vi "Obtain Broadcast Events.vi"(8 "error in":errorcluster, 10 "Create New? (F)":bool) -> (0 "error out":errorcluster, 2 "RT Acquisition Engine Broadcast Events":T1)   [LabVIEW 2021, in "RT Acquisition Engine.lvlib"]
doc: "This VI Obtains/Creates the Broadcast events that will be used for other modules to register to receive messages from the module that owns this VI.\n\n<b>NOTE</b>: The contents of this VI are automatically generated and modified by the <b>Tools > DQMH Consortium > DQMH</b> utilities. Consider using those utilities instead of making your own modifications to this VI.\n_____\nBased on DQMH Project Template 7.0.1.1316."
uses:
  RT Acquisition Engine.lvlib
  Broadcast Events--cluster.ctl
  Did Init Argument--cluster.ctl
  Status Updated Argument--cluster.ctl
  Error Reported Argument--cluster.ctl
  Stop Argument--cluster.ctl
  Get Module Execution Status Argument--cluster.ctl
  RT Connection Status Argument--cluster.ctl
  Hardware Info (Reply Payload)--cluster.ctl
  DO Data's Argument--cluster.ctl
  Host-Control's/DIO Data's from RT.ctl
  AI-Info Argument--cluster.ctl
  Host-Control's/AI-Data from RT.ctl
  Logging Completed Argument--cluster.ctl
panel:
  # "NOTE: The contents of this VI are automatically generated and modified by the Tools > DQMH Consortium > DQMH utilities. Consider using those utilities instead of making your own modifications to this VI."
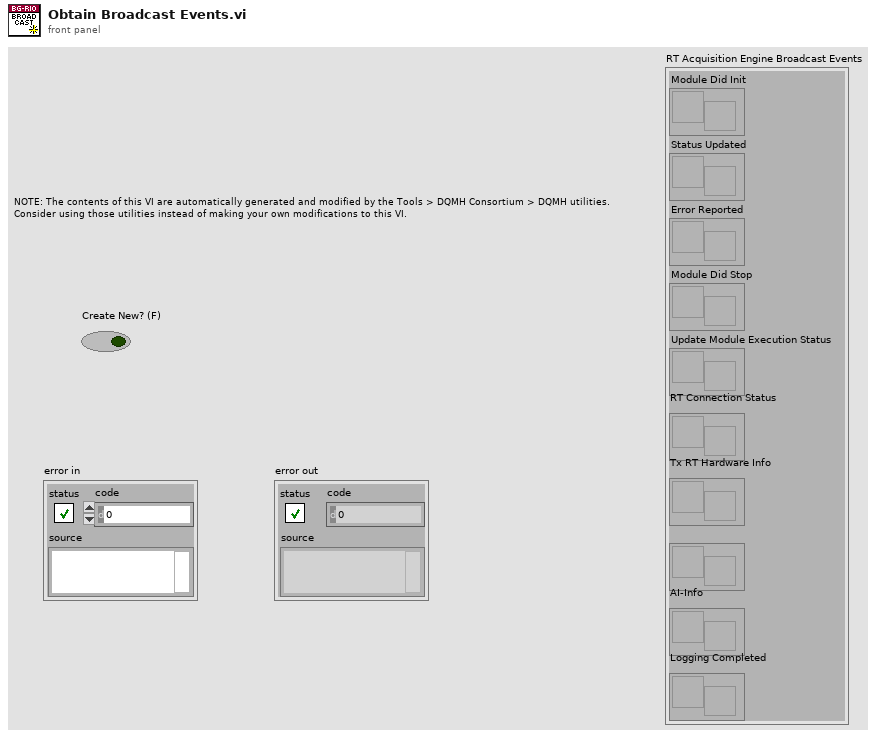
[diagram p1: front panel]
types:
  T1 = typedef "RT Acquisition Engine.lvlib/Broadcast Events--cluster.ctl" = cluster{"Module Did Init":refnum<user-event>, "Status Updated":refnum<user-event>, "Error Reported":refnum<user-event>, "Module Did Stop":refnum<user-event>, "Update Module Execution Status":refnum<user-event>, "RT Connection Status":refnum<user-event>, "Tx RT Hardware Info":refnum<user-event>, "DO Data's":refnum<user-event>, "AI-Info":refnum<user-event>, "Logging Completed":refnum<user-event>}
  T2 = typedef "RT Acquisition Engine.lvlib/Logging Completed Argument--cluster.ctl" = cluster{"Module ID":i32, "Logging Completed?":bool}
  T3 = typedef "RT Acquisition Engine.lvlib/AI-Info Argument--cluster.ctl" = cluster{"Module ID":i32, "AI-Info":T4}
  T4 = typedef "AI-Data from RT.ctl" = cluster{"Channel Name's":string[], "Channel Data's":dbl[], "Date & Time":string}
  T5 = typedef "RT Acquisition Engine.lvlib/DO Data's Argument--cluster.ctl" = cluster{"Module ID":i32, "DO Data's":T6}
  T6 = typedef "DIO Data's from RT.ctl" = cluster{"Channels":string[], "Data":bool[], "Time":string}
  T7 = typedef "RT Acquisition Engine.lvlib/Hardware Info (Reply Payload)--cluster.ctl" = cluster{"Module ID":i32, "Hardware Information":variant, "error":errorcluster}
  T8 = typedef "RT Acquisition Engine.lvlib/RT Connection Status Argument--cluster.ctl" = cluster{"Module ID":i32, "RT Connection Status?":bool}
  T9 = typedef "RT Acquisition Engine.lvlib/Get Module Execution Status Argument--cluster.ctl" = cluster{"Module ID":i32, "Running?":bool}
  T10 = typedef "RT Acquisition Engine.lvlib/Stop Argument--cluster.ctl" = cluster{"Module ID":i32, "Origin":string, "Exit via Stop Module Req?":bool, "Wait for Module to stop?":bool}
  T11 = typedef "RT Acquisition Engine.lvlib/Error Reported Argument--cluster.ctl" = cluster{"Error":errorcluster, "Additional Information":string, "Module ID":i32, "Module Name":string}
  T12 = typedef "RT Acquisition Engine.lvlib/Status Updated Argument--cluster.ctl" = cluster{"Status":string, "Module ID":i32}
  T13 = typedef "RT Acquisition Engine.lvlib/Did Init Argument--cluster.ctl" = cluster{"Init?":bool, "Info":string, "Module ID":i32}
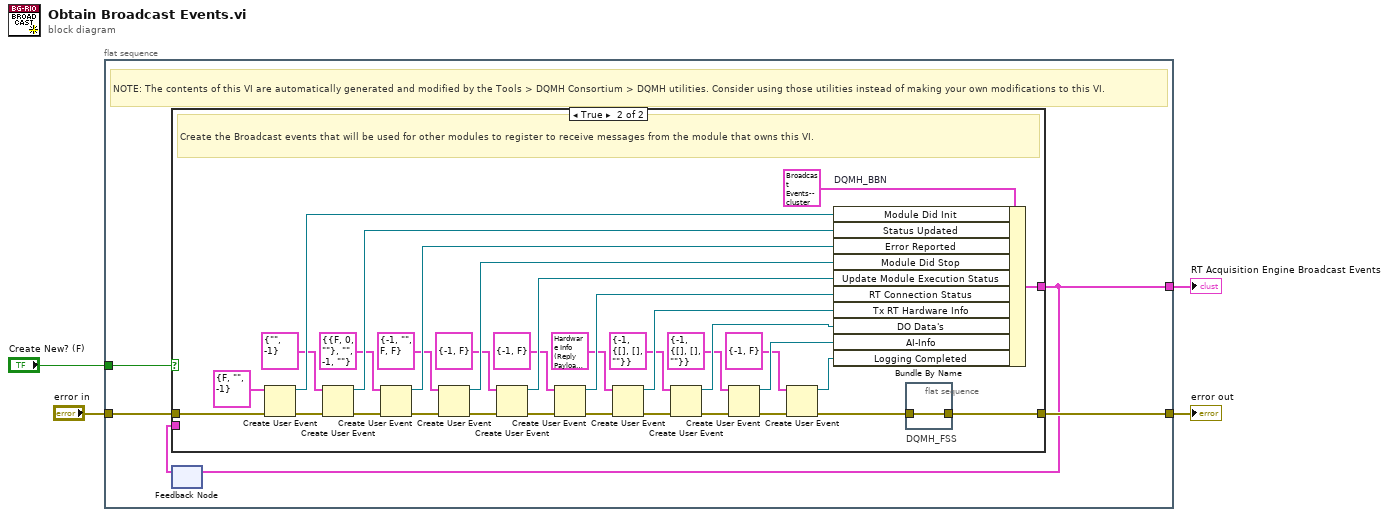
[diagram p0: block diagram]
diagram:
  n1 = flat-sequence {
    tunnel: [w9] -> w4
    tunnel: "error in" -> [w8]
    tunnel: [w6] -> w2
    tunnel: "Create New? (F)" -> [w5]
    frame #0 {
      # "NOTE: The contents of this VI are automatically generated and modified by the Tools > DQMH Consortium > DQMH utilities. Consider using those utilities instead of making your own modifications to this VI."
      n2 = feedback #1() -> (w7:T1)  [unwired: 1 in]
      n3 = case shown="True" w5 {
        tunnel: [w10 w30] -> w9
        tunnel: w8 -> [w10 w45]
        tunnel: [w11 w42] -> w6
        tunnel: w7 -> [w11 _]
        frame False {
          # "Obtain the Broadcast events that were created in a previous call to this VI."
        }
        frame True {
          # "Create the Broadcast events that will be used for other modules to register to receive messages from the module that owns this VI."
          n4 = Create User Event(user event datatype=T13 {"Init?"=FALSE, "Info"="", "Module ID"=-1} ("Did Init Argument"), error in=w45) -> (user event=w43:refnum<user-event>, error out=w40:errorcluster)
          n5 = Create User Event(user event datatype=T12 {"Status"="", "Module ID"=-1} ("Status Updated Argument"), error in=w40) -> (user event=w37:refnum<user-event>, error out=w39:errorcluster)
          n6 = Create User Event(user event datatype=T11 {"Error"={"status"=FALSE, "code"=0, "source"=""}, "Additional Information"="", "Module ID"=-1, "Module Name"=""} ("Error Reported Argument"), error in=w39) -> (user event=w34:refnum<user-event>, error out=w36:errorcluster)
          n7 = Create User Event(user event datatype=T10 {"Module ID"=-1, "Origin"="", "Exit via Stop Module Req?"=FALSE, "Wait for Module to stop?"=FALSE} ("Stop Argument"), error in=w36) -> (user event=w32:refnum<user-event>, error out=w31:errorcluster)
          n8 = Create User Event(user event datatype=T9 {"Module ID"=-1, "Running?"=FALSE} ("Get Module Execution Status Argument"), error in=w31) -> (user event=w28:refnum<user-event>, error out=w29:errorcluster)
          n9 = Create User Event(user event datatype=T8 {"Module ID"=-1, "RT Connection Status?"=FALSE} ("RT Connection Status Argument"), error in=w29) -> (user event=w25:refnum<user-event>, error out=w26:errorcluster)
          n10 = Create User Event(user event datatype=T7 {"Module ID"=-1, "Hardware Information"=variant(cluster{"Serial Hardware Info JSON Format":cluster{"Command":string, "SubCmd":string, "Channel":string[]}, "Hardware Info JSON Format":cluster{"Command":string, "SubCmd":string, "Input":string[], "Output":string[]}, "Hardware Info JSON Format":cluster{"Command":string, "SubCmd":string, "Input":string[], "Output":string[]}, "Ethernet IP Address JSON Format":cluster{"Command":string, "SubCmd":string, "IP":string[]}} {"Serial Hardware Info JSON Format"={"Command"="", "SubCmd"="", "Channel"=[]}, "Hardware Info JSON Format"={"Command"="", "SubCmd"="", "Input"=[], "Output"=[]}, "Hardware Info JSON Format"={"Command"="", "SubCmd"="", "Input"=[], "Output"=[]}, "Ethernet IP Address JSON Format"={"Command"="", "SubCmd"="", "IP"=[]}}), "error"={"status"=FALSE, "code"=0, "source"=""}} ("Hardware Info (Reply Payload)"), error in=w26) -> (user event=w22:refnum<user-event>, error out=w23:errorcluster)
          n11 = Create User Event(user event datatype=T5 {"Module ID"=-1, "DO Data's"={"Channels"=[], "Data"=[], "Time"=""}} ("DO Data's Argument"), error in=w23) -> (user event=w19:refnum<user-event>, error out=w20:errorcluster)
          n12 = Create User Event(user event datatype=T3 {"Module ID"=-1, "AI-Info"={"Channel Name's"=[], "Channel Data's"=[], "Date & Time"=""}} ("AI-Info Argument"), error in=w20) -> (user event=w16:refnum<user-event>, error out=w17:errorcluster)
          n13 = Create User Event(user event datatype=T2 {"Module ID"=-1, "Logging Completed?"=FALSE} ("Logging Completed Argument"), error in=w17) -> (user event=w13:refnum<user-event>, error out=w14:errorcluster)
          n14 = Bundle By Name "DQMH_BBN"(cluster=T1 {"Module Did Init"=refnum, "Status Updated"=refnum, "Error Reported"=refnum, "Module Did Stop"=refnum, "Update Module Execution Status"=refnum, "RT Connection Status"=refnum, "Tx RT Hardware Info"=refnum, "DO Data's"=refnum, "AI-Info"=refnum, "Logging Completed"=refnum} ("output cluster"), "Module Did Init"=w43, "Status Updated"=w37, "Error Reported"=w34, "Module Did Stop"=w32, "Update Module Execution Status"=w28, "RT Connection Status"=w25, "Tx RT Hardware Info"=w22, "DO Data's"=w19, "AI-Info"=w16, "Logging Completed"=w13) -> (w42:T1)
          n15 = flat-sequence "DQMH_FSS" {
            tunnel: w14 -> [w46]
            tunnel: [w46] -> w30
            frame #0 {
            }
          }
        }
      }
      n16 = feedback-in #1(w6) -> ()
    }
  }
  "RT Acquisition Engine Broadcast Events" <- w2
  "error out" <- w4
